vi "ZachArmPosition2.vi"(8 "Manual Position":dbl, 9 "Arm Position":dbl, 11 "User Arm Position":T1) -> (1 "Target Position":dbl, 2 "Motor Speed":dbl)   [LabVIEW 2013]
uses:
  Arm Postions Enum Typedef.ctl
  Arm State Enum Typedef.ctl
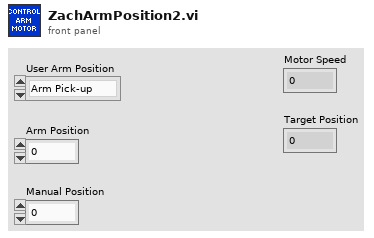
[diagram p1: front panel]
types:
  T1 = typedef "Arm Postions Enum Typedef.ctl" = enum16{"Arm Pick-up", "Idle", "Arm Shoot", "Arm Truss", "Manual"}
  T2 = typedef "Arm State Enum Typedef.ctl" = enum16{"AtPickup", "AtShoot", "AtTruss"}
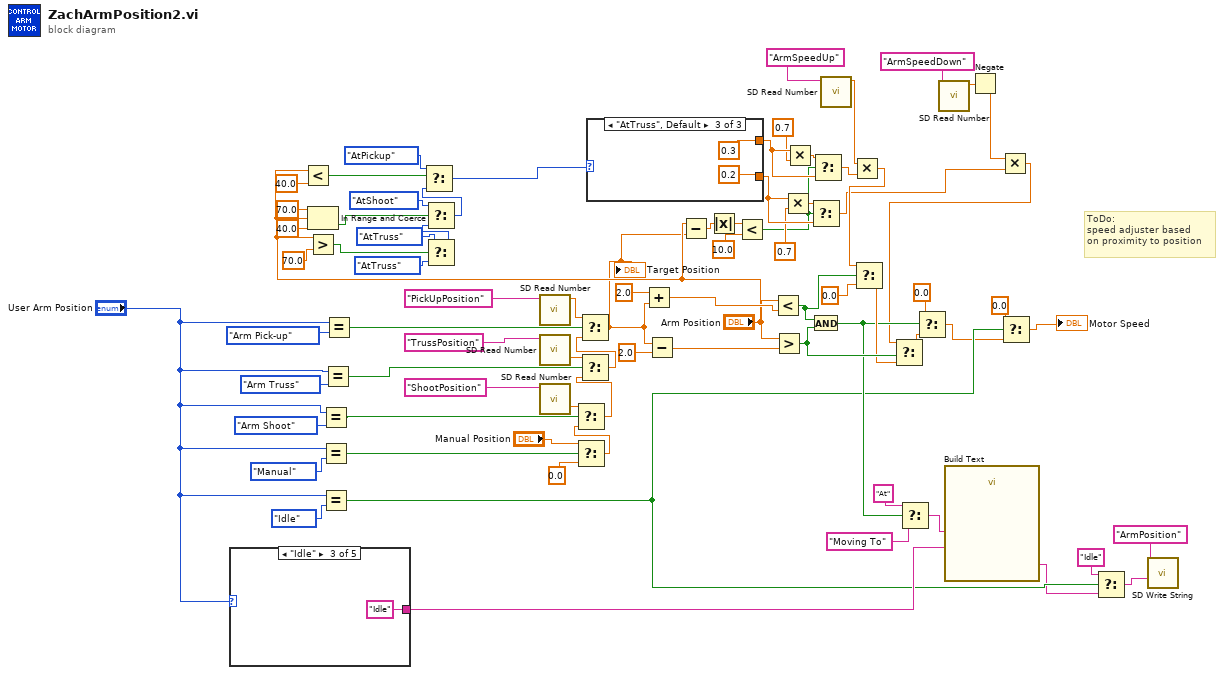
[diagram p0: block diagram]
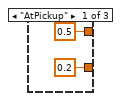
[diagram p2: hidden frame]
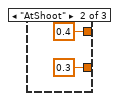
[diagram p3: hidden frame]
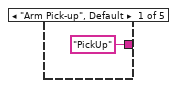
[diagram p4: hidden frame]
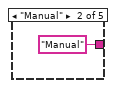
[diagram p5: hidden frame]
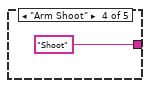
[diagram p6: hidden frame]
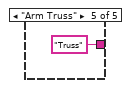
[diagram p7: hidden frame]
diagram:
  # "ToDo:\nspeed adjuster based\non proximity to position"
  n1 = case shown="\"Idle\"" "User Arm Position" {
    tunnel: ["PickUp" "Manual" "Idle" "Shoot" "Truss"] -> w56
    frame "Arm Pick-up", Default {
    }
    frame "Manual" {
    }
    frame "Idle" {
    }
    frame "Arm Shoot" {
    }
    frame "Arm Truss" {
    }
  }
  n2 = Less?(x="Arm Position", y=40.0 ("upper limit")) -> (x < y?=w23:bool)
  n3 = In Range and Coerce(upper limit=70.0, x="Arm Position", lower limit=40.0) -> (In Range?=w24:bool)  [unwired: 1 out]
  n4 = Greater?(x="Arm Position", y=70.0) -> (0:w25:bool)
  n5 = Equal?(x="User Arm Position", y=Arm_Postions_Enum_Typedef."Arm Shoot") -> (x = y?=w66:bool)
  n6 = Equal?(x="User Arm Position", y=Arm_Postions_Enum_Typedef."Manual") -> (x = y?=w40:bool)
  n7 = Equal?(x="User Arm Position", y=Arm_Postions_Enum_Typedef."Idle") -> (x = y?=w34:bool)
  n8 = Equal?(x="User Arm Position", y=Arm_Postions_Enum_Typedef."Arm Truss") -> (x = y?=w67:bool)
  n9 = Equal?(x="User Arm Position", y=Arm_Postions_Enum_Typedef."Arm Pick-up") -> (x = y?=w65:bool)
  n10 = Select(t=Arm_State_Enum_Typedef."AtTruss" ("Arm State"), s=w25, f=Arm_State_Enum_Typedef."AtTruss" ("Arm State")) -> (s? t:f=w22:T2)
  n11 = Select(t=Arm_State_Enum_Typedef."AtShoot" ("Arm State"), s=w24, f=w22) -> (s? t:f=w21:T2)
  n12 = Select(t=Arm_State_Enum_Typedef."AtPickup" ("Arm State"), s=w23, f=w21) -> (s? t:f=w15:T2)
  n13 = call <vilib>:"SD Read Number.vi"("Name"="PickUpPosition" ("Table Prefix")) -> ("Numeric"=w48:dbl)  [unwired: 8 in, 2 out]
  n14 = call <vilib>:"SD Read Number.vi"("Name"="TrussPosition" ("Table Prefix")) -> ("Numeric"=w61:dbl)  [unwired: 8 in, 2 out]
  n15 = call <vilib>:"SD Read Number.vi"("Name"="ShootPosition" ("Table Prefix")) -> ("Numeric"=w60:dbl)  [unwired: 8 in, 2 out]
  n16 = Select(t="Manual Position", s=w40, f=0.0) -> (s? t:f=w42:dbl)
  n17 = Select(t=w60, s=w66, f=w42) -> (s? t:f=w78:dbl)
  n18 = Select(t=w61, s=w67, f=w78) -> (s? t:f=w79:dbl)
  n19 = Select(t=w48, s=w65, f=w79) -> (s? t:f=w10:dbl)
  "Target Position" <- w10
  n20 = case shown="\"AtTruss\", Default" w15 {
    tunnel: [0.5 0.4 0.3] -> w6
    tunnel: [0.2 0.3 0.2] -> w5
    frame "AtPickup" {
    }
    frame "AtShoot" {
    }
    frame "AtTruss", Default {
    }
  }
  n21 = Add(x=2.0, y=w10) -> (x+y=w74:dbl)
  n22 = Subtract(x=w10, y=2.0) -> (x-y=w75:dbl)
  n23 = Subtract(x="Arm Position", y=w10) -> (x-y=w47:dbl)
  n24 = Absolute Value(x=w47) -> (abs(x)=w46:dbl)
  n25 = Less?(x=w46, y=10.0) -> (x < y?=w1:bool)
  n26 = Less?(x="Arm Position", y=w74) -> (x < y?=w73:bool)
  n27 = Greater?(x="Arm Position", y=w75) -> (0:w72:bool)
  n28 = Multiply(x=w5, y=0.7) -> (x*y=w9:dbl)
  n29 = Multiply(x=w6, y=0.7) -> (x*y=w8:dbl)
  n30 = Select(t=w9, s=w1, f=w5) -> (s? t:f=w2:dbl)
  n31 = And(x=w73, y=w72) -> (x .and. y?=w52:bool)
  n32 = Select(t=w8, s=w1, f=w6) -> (s? t:f=w7:dbl)
  n33 = call <vilib>:"SD Read Number.vi"("Name"="ArmSpeedUp") -> ("Numeric"=w29:dbl)  [unwired: 8 in, 2 out]
  n34 = Multiply(x=w29, y=w7) -> (x*y=w26:dbl)
  n35 = Select(t=w26, s=w73, f=0.0) -> (s? t:f=w71:dbl)
  n36 = Select(t="At" ("Name"), s=w52, f="Moving To" ("Name")) -> (s? t:f=w55:string)
  n37 = call <vilib>:"SD Read Number.vi"("Name"="ArmSpeedDown") -> ("Numeric"=w44:dbl)  [unwired: 8 in, 2 out]
  n38 = call "Build Text"("Moving"=w55, "Place"=w56) -> ("Result"=w31:string)  [unwired: 12 in, 1 out]
  n39 = Negate(x=w44) -> (-x=w28:dbl)
  n40 = Multiply(x=w28, y=w2) -> (x*y=w27:dbl)
  n41 = Select(t=w27, s=w72, f=w71) -> (s? t:f=w70:dbl)
  n42 = Select(t=0.0, s=w52, f=w70) -> (s? t:f=w33:dbl)
  n43 = Select(t=0.0, s=w34, f=w33) -> (s? t:f=→"Motor Speed":dbl)
  n44 = Select(t="Idle" ("f"), s=w34, f=w31) -> (s? t:f=w35:string)
  n45 = call <vilib>:"SD Write String.vi"("String"=w35, "Name"="ArmPosition") -> ()  [unwired: 8 in, 2 out]
